vi "example tcp read.vi"() -> ()   [LabVIEW 2013]
panel:
  out "ErrorOut":errorcluster
  out "TCPData":string[](array[string])
  in  "stop":bool
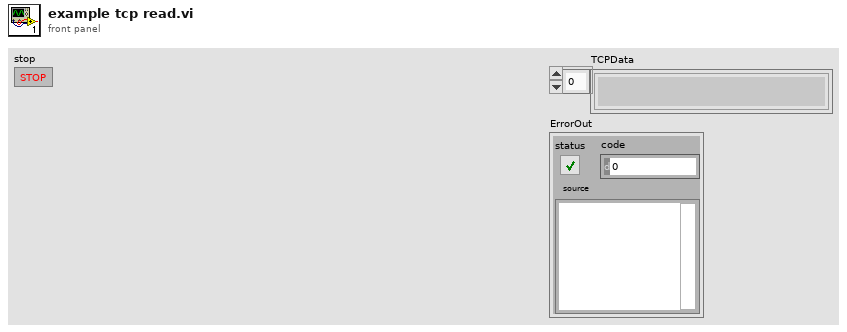
[diagram p1: front panel]
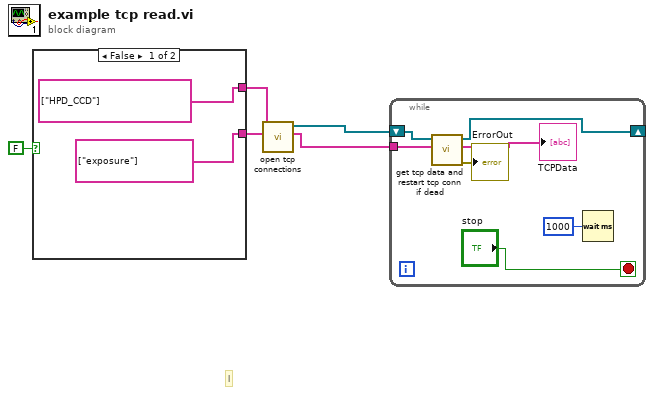
[diagram p0: block diagram]
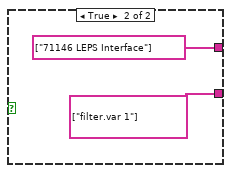
[diagram p2: hidden frame]
diagram:
  # "l"
  n1 = case shown="False" FALSE {
    tunnel: [string[] ["exposure"] ("variables to get data from") string[] ["filter.var 1"] ("variables to get data from")] -> w5
    tunnel: [string[] ["HPD_CCD"] ("devices to get data from") string[] ["71146 LEPS Interface"] ("devices to get data from")] -> w3
    frame False {
    }
    frame True {
    }
  }
  n2 = call "open tcp connections.vi"("variables to get data from"=w5, "devices to get data from"=w3) -> ("subscribe messages\nfor process vis"=w4:string[], "tcp connections"=w2:refnum<k5>[])  [unwired: 8 in]
  n3 = while {
    tunnel: w4 -> [w16]
    shift-right: [w12] -> _
    shift-left: w2 -> [w11]
    stop <- "stop" stop-if-true
    n4 = call "get tcp data and restart tcp conn if dead.vi"("Subscribe Messages"=w16, "TCPRefs in"=w11) -> ("ErrorOut"=→"ErrorOut":errorcluster, "TCPData"=→"TCPData":string[], "TCPRefs out"=w12:refnum<k5>[])  [unwired: 7 in]
    n5 = Wait (ms)(milliseconds to wait=u32 1000) -> ()  [unwired: 1 out]
  }
